vi "Parse sender and receivers.vi"(11 "String":string) -> (2 "Receivers":string[](array[string]), 3 "Sender":string)   [LabVIEW 2021, in "Module.lvclass"]
uses:
  Module.lvclass
  Helpers/Helpers.lvlib
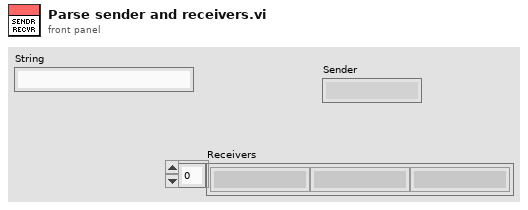
[diagram p1: front panel]
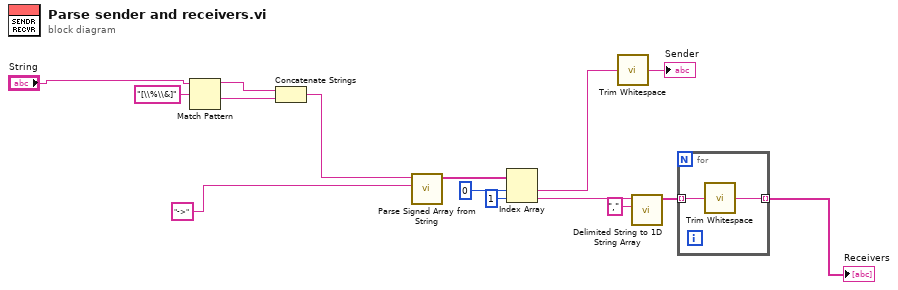
[diagram p0: block diagram]
diagram:
  n1 = Match Pattern(string="String", regular expression="[\\%\\&]") -> (before substring=w1:string, after substring=w3:string)  [unwired: 1 in, 2 out]
  n2 = Concatenate Strings(w1, w3) -> (w2:string)
  n3 = call "Parse Signed Array from String.vi"("Delimiter regex"="->", "Input"=w2) -> ("Parsed Array"=w8:string[])  [unwired: 8 in, 1 out]
  n4 = Index Array(array=w8, index #1=0 ("index"), index #2=1 ("index")) -> (element #1=w15:string, element #2=w10:string)
  n5 = call <vilib>:"Trim Whitespace.vi"("string"=w15) -> ("trimmed string"=→"Sender":string)  [unwired: 1 in]
  n6 = call <vilib>:"Delimited String to 1D String Array.vi"("delimiter"=",", "delimited string"=w10) -> ("string array"=w12:string[])  [unwired: 9 in]
  n7 = for {
    tunnel: w12 -> [w17] mode=indexing
    tunnel: [w16] -> w13 mode=indexing
    n8 = call <vilib>:"Trim Whitespace.vi"("string"=w17) -> ("trimmed string"=w16:string)  [unwired: 1 in]
  }
  "Receivers" <- w13
